vi "Acquiring.vi"(8 "error in (no error)":errorcluster, 11 "Father Of All Detectors in":refnum<class "Father Of All Detectors.lvclass">) -> (0 "error out":errorcluster, 2 "Ready to Save Data?":bool, 3 "Father Of All Detectors out":refnum<class "Father Of All Detectors.lvclass">)   [LabVIEW 2026, in "TALOS.lvlib" / "Father Of All Detectors.lvlib" / "Father Of All Detectors.lvclass"]
doc: "Use \"Ready to Save Data?\" to indicate if the data acquisition is terminated (and therefore is possible to move to Save Data), or if it is not terminated, and therefore is needed to come back to Acquiring (this VI)."
uses:
  Father Of All Detectors.lvclass
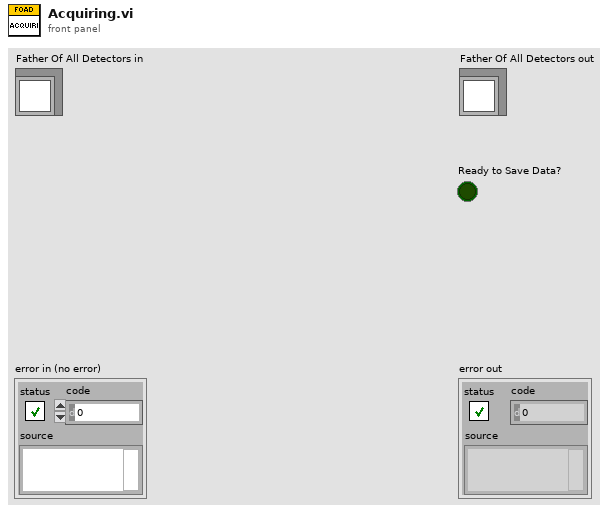
[diagram p1: front panel]
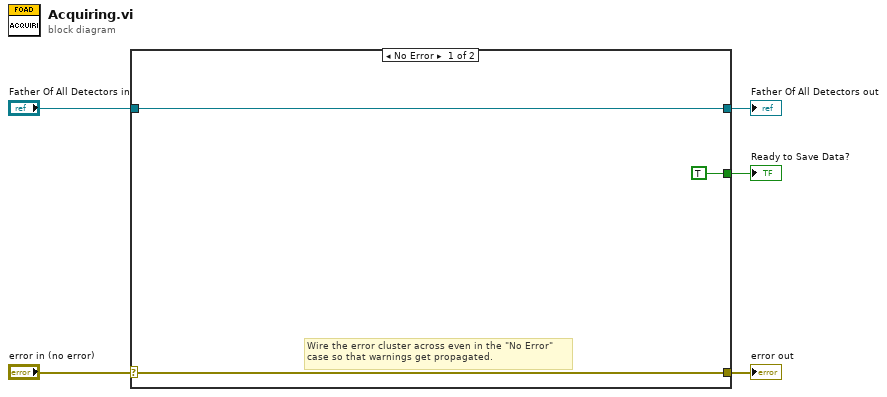
[diagram p0: block diagram]
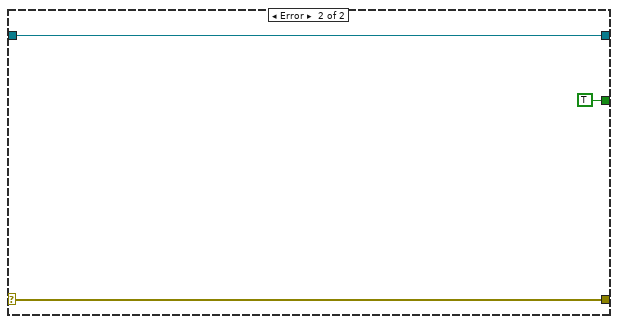
[diagram p2: hidden frame]
diagram:
  n1 = case shown="No Error" "error in (no error)" {
    selector: "error in (no error)" -> [w7 w11]
    tunnel: [w7 w11] -> w4
    tunnel: [w8 w10] -> w2
    tunnel: "Father Of All Detectors in" -> [w8 w10]
    tunnel: [TRUE TRUE] -> w1
    frame No Error {
      # "Wire the error cluster across even in the \"No Error\"\ncase so that warnings get propagated."
    }
    frame Error {
    }
  }
  "error out" <- w4
  "Father Of All Detectors out" <- w2
  "Ready to Save Data?" <- w1
